vi "Save Updated Project.vi"(8 "error in (no error)":errorcluster, 11 "Project in":refnum<class "Project.lvclass">) -> (0 "error out":errorcluster, 3 "Project out":refnum<class "Project.lvclass">)   [LabVIEW 2015, in "Project.lvclass"]
uses:
  Project.lvclass
  Project.lvclass/Project.ctl
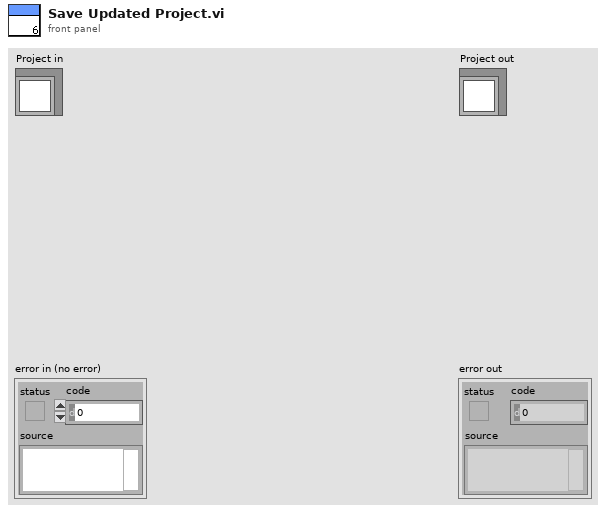
[diagram p1: front panel]
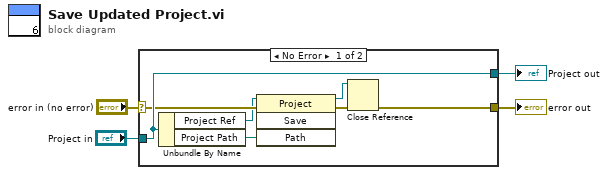
[diagram p0: block diagram]
diagram:
  n1 = case shown="No Error" "error in (no error)" {
    selector: "error in (no error)" -> [w7 w13]
    tunnel: [w6 w13] -> w3
    tunnel: [w8 w12] -> w1
    tunnel: "Project in" -> [w8 w12]
    frame No Error {
      n2 = Unbundle By Name(w8) -> ("Project Ref"=w5:refnum<vi>, "Project Path"=w9:path)
      n3 = invoke class="Project" method="Save"(reference=w5, error in=w7, "Path"=w9) -> (reference out=w11:refnum<vi>, error out=w10:errorcluster)  [unwired: 1 in, 2 out]
      n4 = Close Reference(reference=w11, error in (no error)=w10) -> (error out=w6:errorcluster)
    }
    frame Error {
    }
  }
  "error out" <- w3
  "Project out" <- w1
